vi "GetHelp.vi"(11 "AddNum in":refnum<class "AddTwoNumbers.lvclass">) -> (2 "Help":string, 3 "AddNum out":refnum<class "AddTwoNumbers.lvclass">)   [LabVIEW 2014, in "AddTwoNumbers.lvclass"]
doc: "This operation vi returns help for AddTwoNumbers operation."
uses:
  AddTwoNumbers.lvclass
panel:
  in  "Help":string="This operation adds two I32 numbers.\nSpecify number to add as command line parameter to the VI.\nExample: LabVIEWCLI -OperationName AddNum 100 200"
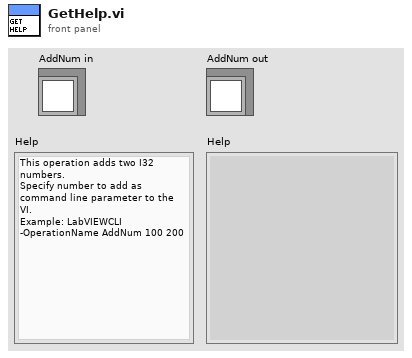
[diagram p1: front panel]
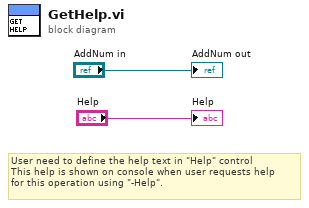
[diagram p0: block diagram]
diagram:
  # "User need to define the help text in \"Help\" control\nThis help is shown on console when user requests help\nfor this operation using \"-Help\"."
  "AddNum out" <- "AddNum in"
  "Help" <- "Help"
